vi "Default.vi"(8 "error in (no error)":errorcluster, 11 "UIStep in":refnum<class "UIStep.lvclass">) -> (0 "error out":errorcluster, 3 "UIStep out":refnum<class "UIStep.lvclass">)   [LabVIEW 2015, in "UIStep.lvclass"]
uses:
  UIStep.lvclass
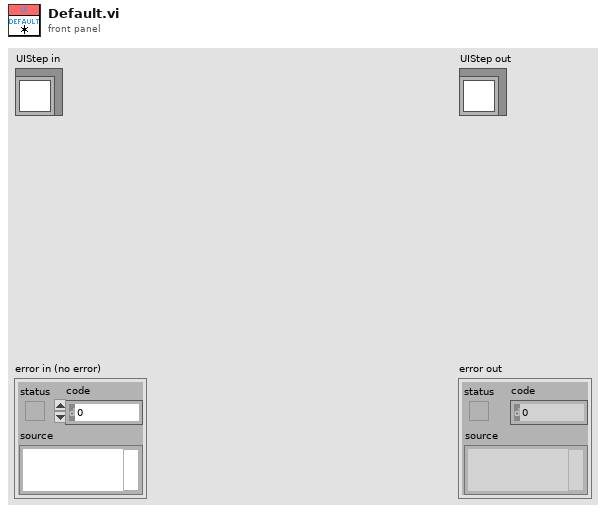
[diagram p1: front panel]
types:
  T1 = cluster{"Button1":cluster{"Label":string, "Size":dbl, "TextColor":u32, "BGColor":u32, "Bold":bool}, "Button2":cluster{"Label":string, "Size":dbl, "TextColor":u32, "BGColor":u32, "Bold":bool}}
  T2 = cluster{"Font":string, "Size":dbl, "Justification":u16, "TextColor":u32, "BGColor":u32, bool}
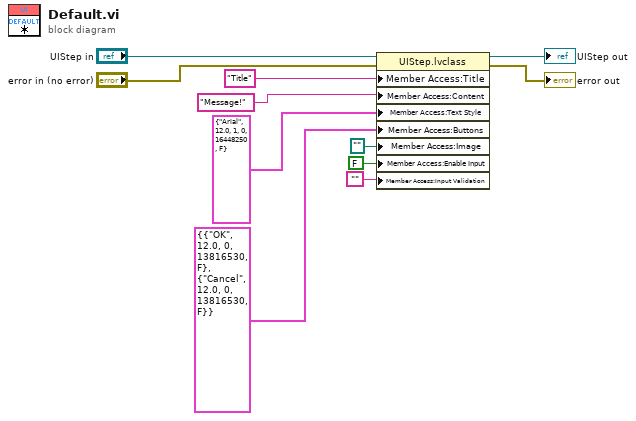
[diagram p0: block diagram]
diagram:
  n1 = property class="UIStep.lvclass"(reference="UIStep in", error in="error in (no error)", "Member Access:Title"="Title" ("Title"), "Member Access:Content"="Message!" ("Content"), "Member Access:Text Style"=T2 {"Font"="Arial", "Size"=12.0, "Justification"=1, "TextColor"=0, "BGColor"=16448250, FALSE} ("Text Style"), "Member Access:Buttons"=T1 {"Button1"={"Label"="OK", "Size"=12.0, "TextColor"=0, "BGColor"=13816530, "Bold"=FALSE}, "Button2"={"Label"="Cancel", "Size"=12.0, "TextColor"=0, "BGColor"=13816530, "Bold"=FALSE}} ("Buttons"), "Member Access:Image"=path "", "Member Access:Enable Input"=FALSE ("Enable Input"), "Member Access:Input Validation"="") -> (reference out=→"UIStep out":refnum<class "UIStep.lvclass">, error out=→"error out":errorcluster)
